vi "octave_index.vi"(8 "error in (no error)":errorcluster, 10 "Octave 2":T1, 11 "Octave":T1) -> (0 "error out":errorcluster, 1 "min index(es)":i32, 2 "max index(es)":i32, 3 "Is key pressed?":bool)   [LabVIEW 2024]
doc: "dokumwentacja"
uses:
  controls/#typedef_octave.ctl
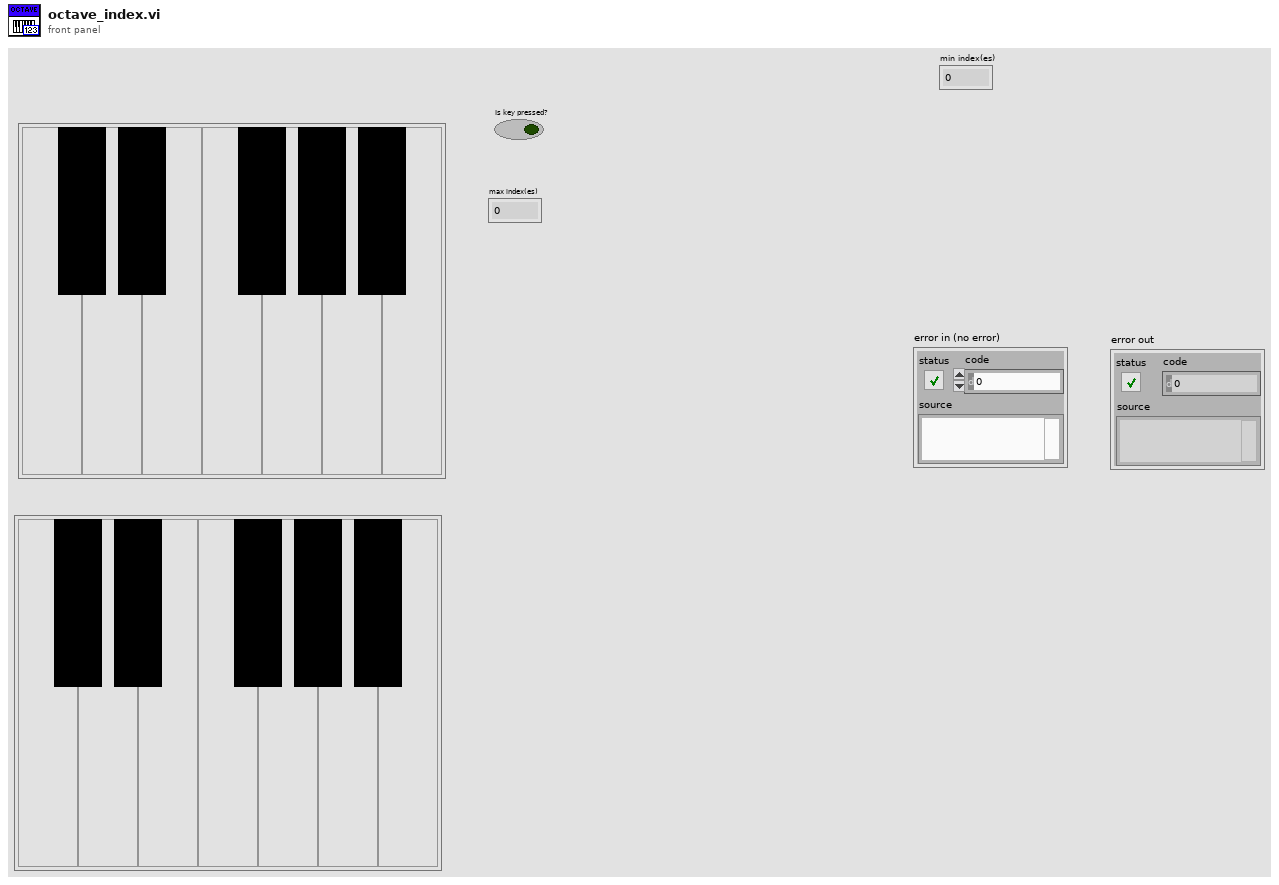
[diagram p1: front panel]
types:
  T1 = typedef "#typedef_octave.ctl" = cluster{"C":bool, "D":bool, "E":bool, "F":bool, "G":bool, "C#":bool, "D#":bool, "A":bool, "G#":bool, "B":bool, "F#":bool, "Bb":bool}
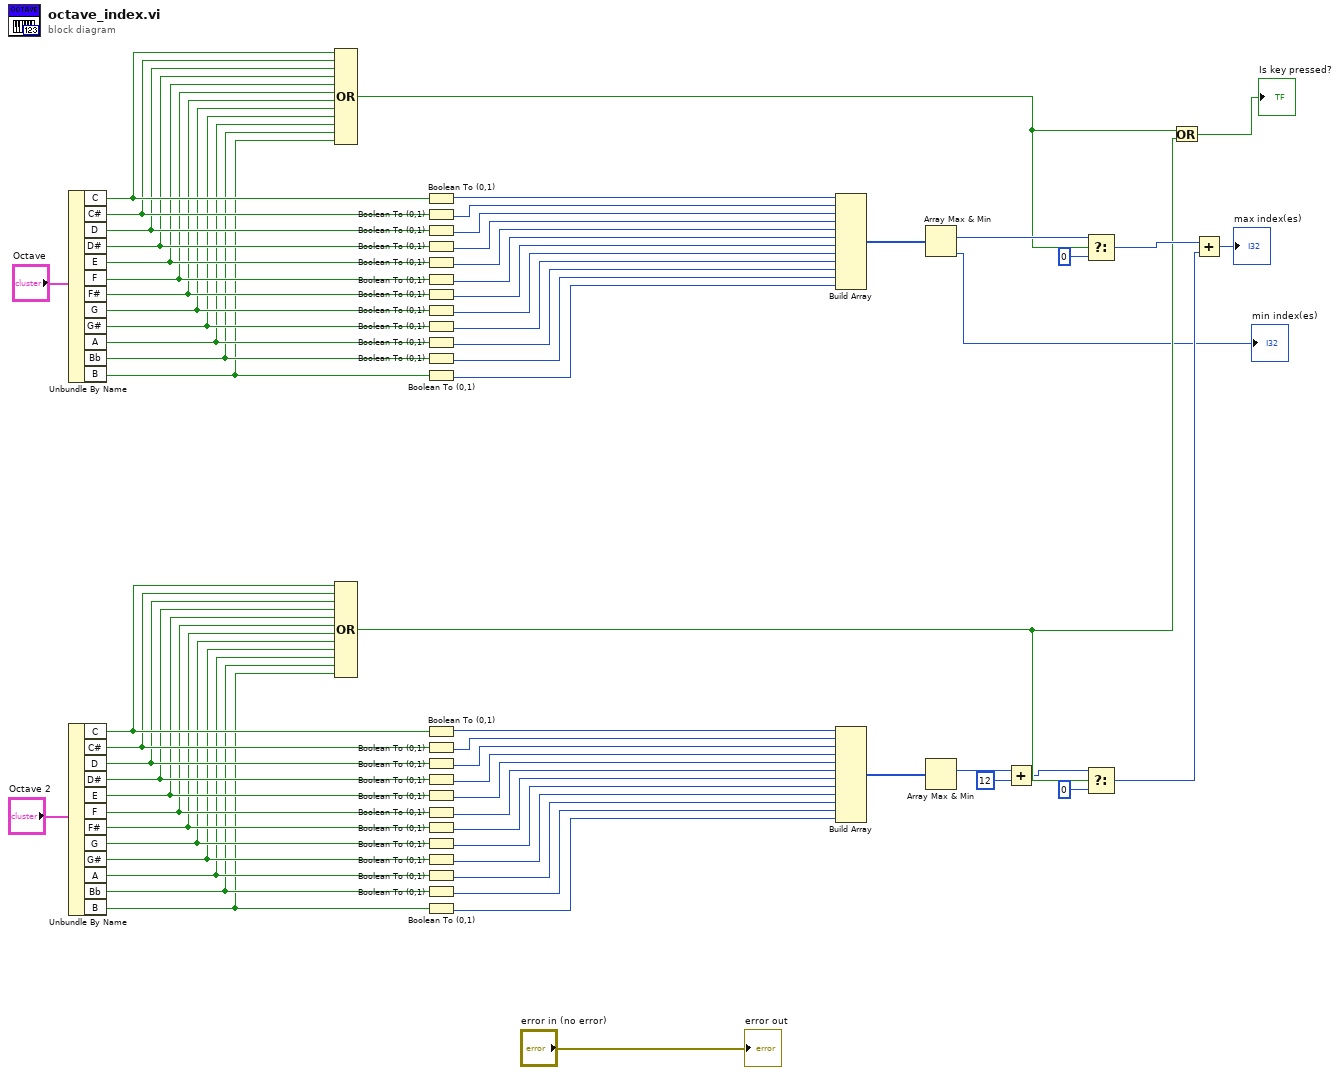
[diagram p0: block diagram]
diagram:
  n1 = Unbundle By Name("Octave") -> ("C"=w63:bool, "C#"=w62:bool, "D"=w61:bool, "D#"=w60:bool, "E"=w59:bool, "F"=w58:bool, "F#"=w57:bool, "G"=w56:bool, "G#"=w55:bool, "A"=w54:bool, "Bb"=w53:bool, "B"=w52:bool)
  n2 = Unbundle By Name("Octave 2") -> ("C"=w34:bool, "C#"=w33:bool, "D"=w32:bool, "D#"=w31:bool, "E"=w30:bool, "F"=w29:bool, "F#"=w28:bool, "G"=w27:bool, "G#"=w26:bool, "A"=w25:bool, "Bb"=w24:bool, "B"=w23:bool)
  n3 = Compound Arithmetic op=OR(w63, w62, w61, w60, w59, w58, w57, w56, w55, w54, w53, w52) -> (w8:bool)
  n4 = Compound Arithmetic op=OR(w34, w33, w32, w31, w30, w29, w28, w27, w26, w25, w24, w23) -> (w7:bool)
  n5 = Boolean To (0,1)(Boolean=w63) -> (0, 1=w66:i16)
  n6 = Boolean To (0,1)(Boolean=w62) -> (0, 1=w65:i16)
  n7 = Boolean To (0,1)(Boolean=w61) -> (0, 1=w64:i16)
  n8 = Boolean To (0,1)(Boolean=w60) -> (0, 1=w51:i16)
  n9 = Boolean To (0,1)(Boolean=w59) -> (0, 1=w50:i16)
  n10 = Boolean To (0,1)(Boolean=w58) -> (0, 1=w49:i16)
  n11 = Boolean To (0,1)(Boolean=w57) -> (0, 1=w48:i16)
  n12 = Boolean To (0,1)(Boolean=w56) -> (0, 1=w47:i16)
  n13 = Boolean To (0,1)(Boolean=w55) -> (0, 1=w46:i16)
  n14 = Boolean To (0,1)(Boolean=w54) -> (0, 1=w45:i16)
  n15 = Boolean To (0,1)(Boolean=w53) -> (0, 1=w44:i16)
  n16 = Boolean To (0,1)(Boolean=w52) -> (0, 1=w43:i16)
  n17 = Boolean To (0,1)(Boolean=w34) -> (0, 1=w37:i16)
  n18 = Boolean To (0,1)(Boolean=w33) -> (0, 1=w36:i16)
  n19 = Boolean To (0,1)(Boolean=w32) -> (0, 1=w35:i16)
  n20 = Boolean To (0,1)(Boolean=w31) -> (0, 1=w22:i16)
  n21 = Boolean To (0,1)(Boolean=w30) -> (0, 1=w21:i16)
  n22 = Boolean To (0,1)(Boolean=w29) -> (0, 1=w20:i16)
  n23 = Boolean To (0,1)(Boolean=w28) -> (0, 1=w19:i16)
  n24 = Boolean To (0,1)(Boolean=w27) -> (0, 1=w18:i16)
  n25 = Boolean To (0,1)(Boolean=w26) -> (0, 1=w17:i16)
  n26 = Boolean To (0,1)(Boolean=w25) -> (0, 1=w16:i16)
  n27 = Boolean To (0,1)(Boolean=w24) -> (0, 1=w15:i16)
  n28 = Boolean To (0,1)(Boolean=w23) -> (0, 1=w14:i16)
  n29 = Build Array(w66, w65, w64, w51, w50, w49, w48, w47, w46, w45, w44, w43) -> (w42:i16[])
  n30 = Build Array(w37, w36, w35, w22, w21, w20, w19, w18, w17, w16, w15, w14) -> (w13:i16[])
  n31 = Array Max & Min(array=w42) -> (max index (indices)=w39:i32, min index (indices)=→"min index(es)":i32)  [unwired: 2 out]
  n32 = Array Max & Min(array=w13) -> (max index (indices)=w12:i32)  [unwired: 3 out]
  n33 = Add(x=w12, y=12) -> (x+y=w4:i32)
  n34 = Select(t=w39, s=w8, f=0) -> (s? t:f=w41:i32)
  n35 = Select(t=w4, s=w7, f=0) -> (s? t:f=w9:i32)
  n36 = Or(x=w8, y=w7) -> (x .or. y?=→"Is key pressed?":bool)
  n37 = Add(x=w41, y=w9) -> (x+y=→"max index(es)":i32)
  "error out" <- "error in (no error)"
